vi "yearlyCheckRMR.vi"(0 "reference in":refnum<class "Notification Controller.lvclass">, 5 "dateString":string, 11 "error in (no error)":errorcluster) -> (4 "reference out":refnum<class "Notification Controller.lvclass">, 10 "send?":bool, 15 "error out":errorcluster)   [LabVIEW 2016, in "Notification Controller.lvclass"]
uses:
  Notification Controller.lvclass
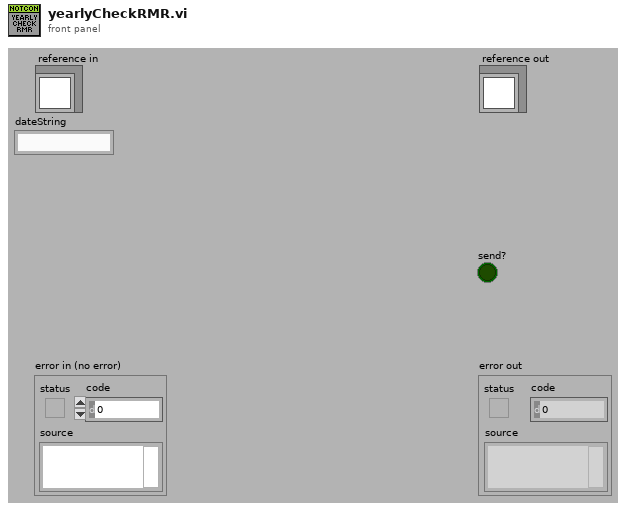
[diagram p1: front panel]
types:
  T1 = cluster{"second":i32, "minute":i32, "hour":i32, "day of month":i32, "month":i32, "year":i32, "day of week":i32, "day of year":i32, "is DST":i32}
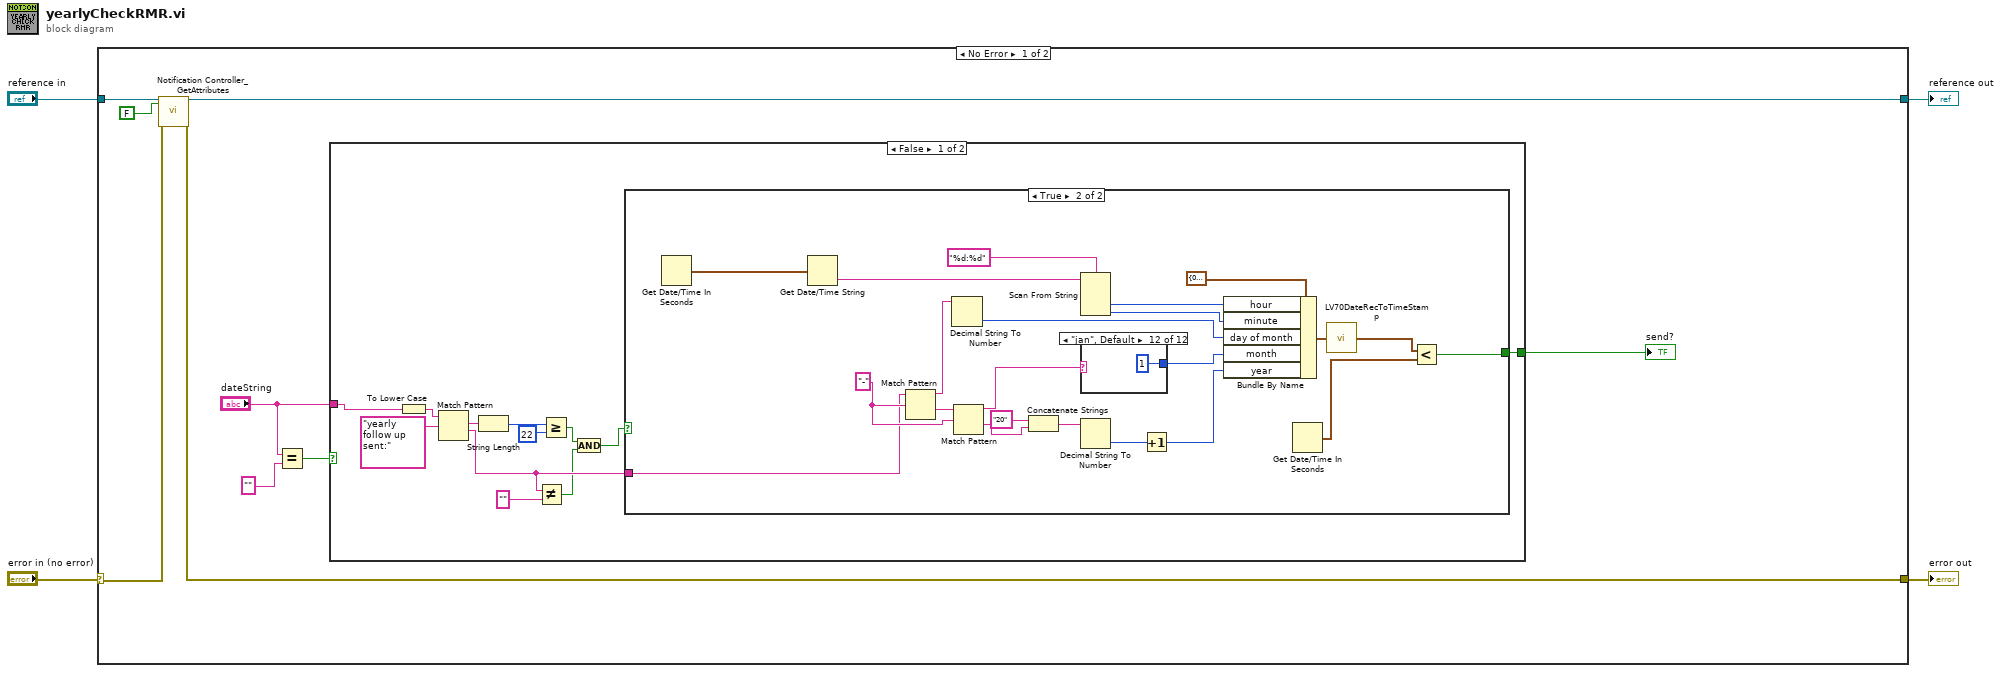
[diagram p0: block diagram]
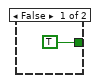
[diagram p2: hidden frame]
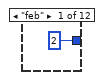
[diagram p3: hidden frame]
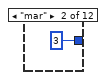
[diagram p4: hidden frame]
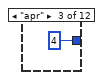
[diagram p5: hidden frame]
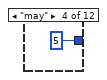
[diagram p6: hidden frame]
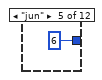
[diagram p7: hidden frame]
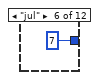
[diagram p8: hidden frame]
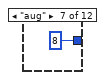
[diagram p9: hidden frame]
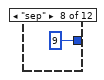
[diagram p10: hidden frame]
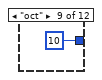
[diagram p11: hidden frame]
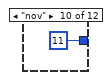
[diagram p12: hidden frame]
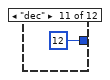
[diagram p13: hidden frame]
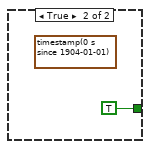
[diagram p14: hidden frame]
diagram:
  n1 = case shown="No Error" "error in (no error)" {
    selector: "error in (no error)" -> [w11 w63]
    tunnel: [w9 w63] -> w3
    tunnel: [w10 w62] -> w1
    tunnel: "reference in" -> [w13 w62]
    frame No Error {
      n2 = call "Notification Controller_GetAttributes.vi"("reference in"=w13, "return data? (T)"=FALSE, "error in (no error)"=w11) -> ("reference out"=w10:refnum<class "Notification Controller.lvclass">, "error out"=w9:errorcluster)  [unwired: 13 in, 2 out]
      n3 = Equal?(x="dateString", y="") -> (x = y?=w5:bool)
      n4 = case shown="False" w5 {
        tunnel: [w25 TRUE] -> w7
        tunnel: "dateString" -> [w19 _]
        frame False {
          n5 = To Lower Case(string=w19) -> (all lower case string=w24:string)
          n6 = Match Pattern(string=w24, regular expression="yearly follow up sent:") -> (match substring=w22:string, after substring=w18:string)  [unwired: 1 in, 2 out]
          n7 = String Length(string=w22) -> (length=w21:i32)
          n8 = Not Equal?(x=w18, y="") -> (x != y?=w15:bool)
          n9 = Greater Or Equal?(x=w21, y=22) -> (x >= y?=w16:bool)
          n10 = And(x=w16, y=w15) -> (x .and. y?=w14:bool)
          n11 = case shown="True" w14 {
            tunnel: [TRUE w30] -> w25
            tunnel: w18 -> [_ w34]
            frame False {
            }
            frame True {
              w39 = "-" ("regular expression")
              n12 = Get Date/Time In Seconds() -> (seconds since 1Jan1904=w48:timestamp)
              n13 = Get Date/Time String(seconds (now)=w48) -> (time string=w42:string)  [unwired: 3 out]
              n14 = Match Pattern(string=w34, regular expression=w39) -> (before substring=w37:string, after substring=w36:string)  [unwired: 1 in, 2 out]
              n15 = Decimal String To Number(string=w37) -> (number=w38:i32)  [unwired: 2 in, 1 out]
              n16 = Match Pattern(string=w36, regular expression=w39) -> (before substring=w41:string, after substring=w27:string)  [unwired: 1 in, 2 out]
              n17 = Concatenate Strings("20" ("string"), w27) -> (w29:string)
              n18 = Scan From String "Scan From String"(format string="%d:%d", input string=w42) -> (output 1=w44:i32, output 2=w43:i32)  [unwired: 4 in, 3 out]
              n19 = case shown="\"jan\", Default" w41 {
                tunnel: [2 ("month") 3 ("month") 4 ("month") 5 ("month") 6 ("month") 7 ("month") 8 ("month") 9 ("month") 10 ("month") 11 ("month") 12 ("month") 1 ("month")] -> w40
                frame "feb" {
                }
                frame "mar" {
                }
                frame "apr" {
                }
                frame "may" {
                }
                frame "jun" {
                }
                frame "jul" {
                }
                frame "aug" {
                }
                frame "sep" {
                }
                frame "oct" {
                }
                frame "nov" {
                }
                frame "dec" {
                }
                frame "jan", Default {
                }
              }
              n20 = Decimal String To Number(string=w29) -> (number=w35:i32)  [unwired: 2 in, 1 out]
              n21 = Increment(x=w35) -> (x+1=w33:i32)
              n22 = Bundle By Name(cluster=T1 {"second"=0, "minute"=0, "hour"=0, "day of month"=0, "month"=0, "year"=0, "day of week"=0, "day of year"=0, "is DST"=0} ("date time rec"), "hour"=w44, "minute"=w43, "day of month"=w38, "month"=w40, "year"=w33) -> (w45:T1)
              n23 = Get Date/Time In Seconds() -> (seconds since 1Jan1904=w31:timestamp)
              n24 = call <vilib>:"LV70DateRecToTimeStamp.vi"("date time rec"=w45) -> ("Time Stamp"=w32:timestamp)
              n25 = Less?(x=w32, y=w31) -> (x < y?=w30:bool)
            }
          }
        }
        frame True {
          (unwired) timestamp(0 s since 1904-01-01) ("Time Stamp")
        }
      }
      "send?" <- w7
    }
    frame Error {
    }
  }
  "error out" <- w3
  "reference out" <- w1
